vi "ReadState.vi"(1 "Input Address":string) -> (0 "Output":i32)   [LabVIEW 2012]
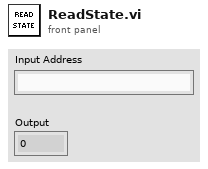
[diagram p1: front panel]
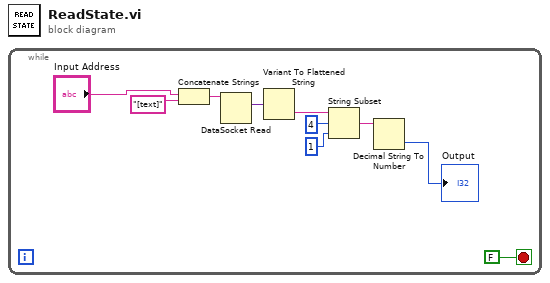
[diagram p0: block diagram]
diagram:
  n1 = while {
    stop <- FALSE stop-if-true
    n2 = Concatenate Strings("Input Address", "[text]" ("string")) -> (w9:string)
    n3 = DataSocket Read(11:w9) -> (2:w8:variant)  [unwired: 4 in, 6 out]
    n4 = Variant To Flattened String(Variant=w8) -> (data string=w4:string)  [unwired: 1 out]
    n5 = String Subset(string=w4, offset (0)=4, length (rest)=1 ("length (rest)")) -> (substring=w5:string)
    n6 = Decimal String To Number(string=w5) -> (number=→"Output":i32)  [unwired: 2 in, 1 out]
  }
